vi "Graph_Settings.vi"() -> ()   [LabVIEW 2018]
uses:
  GraphSettings/GraphSettings_STM.ctl
  GraphSettings/GraphSettings_ITEM.ctl
  CTL/STM GRAPH.ctl
  CTL/Graph settings.ctl
  CTL/Line.ctl
  View.ctl
  <vilib>/Utility/miscctls.llb/LVComboBoxStrsAndValuesArrayTypeDef.ctl
  STM/Grafic/MOKO_Grafic_STM.ctl
  STM/Grafic/MOKO_Grafic_ITEM.ctl
panel:
  in  "Choice Line":string(combo) caption="Combo Box"
  in  "Color Box":u32(colorbox)
  in  "Delete":bool
  in  "Add Line":bool
  in  "Change Line":bool
  in  "Line":T1 {"Color" format="%x"}
  in  "Close":bool
  out "Flat UI Titlebar":bool
  in  "Settings":enum32{"Line", "Data"}(tab)
  in  "STM Graph":T3={"Graph settings"={"Axis X Min"=0.0, "Axis X Name"="", "Axis X Max"=0.0, "Axis Y Min"=0.0, " Axis Y Name"="", "Axis Y Max"=1.0, "Autoscale"=enum."Yes", "Choice Line"=1.0}, "Lines"=[], "Data"=""} {"Lines"."Color" format="%x"}
  out "Graph_Setting":refnum<queue>
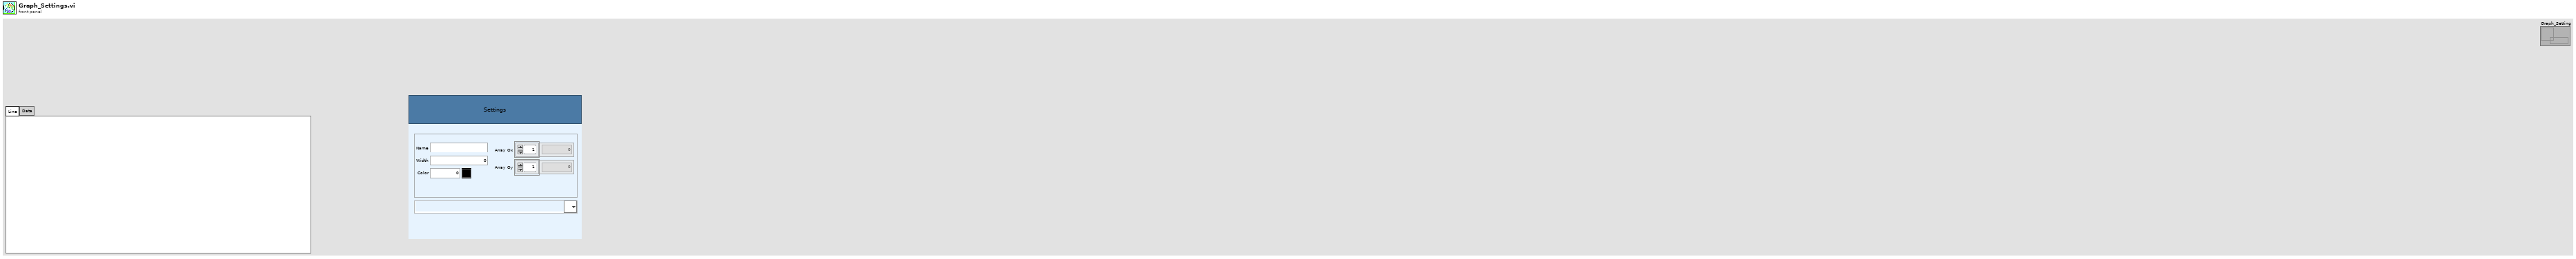
[diagram p1: front panel]
types:
  T1 = typedef "Line.ctl" = cluster{"Width":dbl, "Color":i64, "Array Oy":dbl[], "Array Ox":dbl[], "Name":string, "Plot Visible":T2}
  T2 = typedef "View.ctl" = bool
  T3 = typedef "STM GRAPH.ctl" = cluster{"Graph settings":T4, "Lines":T1[], "Data":string}
  T4 = typedef "Graph settings.ctl" = cluster{"Axis X Min":dbl, "Axis X Name":string, "Axis X Max":dbl, "Axis Y Min":dbl, " Axis Y Name":string, "Axis Y Max":dbl, "Autoscale":enum16{"Yes", "No", "Only Oy", "Only Ox"}, "Choice Line":dbl}
  T5 = typedef "GraphSettings_STM.ctl" = cluster{"main stm":T6, "STM Graph":T3}
  T6 = typedef "GraphSettings_ITEM.ctl" = enum16{"idle", "init", "close", "_____ GRAPH STATE_____ ", "Receive Data", "Send Data", "Change Line", "Delete Line", "Add Line", "Find Max", "Change Color", "Choice Line"}
  T7 = typedef "LVComboBoxStrsAndValuesArrayTypeDef.ctl" = cluster{"String":string, "Value":string}[]
  T8 = typedef "MOKO_Grafic_STM.ctl" = cluster{"main stm":T9, "STM Graph":T3}
  T9 = typedef "MOKO_Grafic_ITEM.ctl" = enum16{"idle", "init", "_____ GRAPH STATE_____ ", "Legend", "Write Graph", "Clear Graph", "close", "Screenshot", "Change Line", "Add Line", "Parse String In", "Add Data", "Change Data", "Graph Settings", "Get Graph Appearance", "Set Graph Appearance", "Delete Data", "Delete Line", "Choose ActPlot", "Set Line Settings", "Increment Smth", "ReWrite Graph", "Autoscale", "Set Autoscale", "Hide Line", "Get Hide Line", "Hide Data", "Show Line", "Get Show Line", "Show Data", "Choose Line", "Change Combo Box", "Send Data", "Receive Data", "Choice Line", "Change Lines", "_____ LED STATE_____ ", "Led Off"}
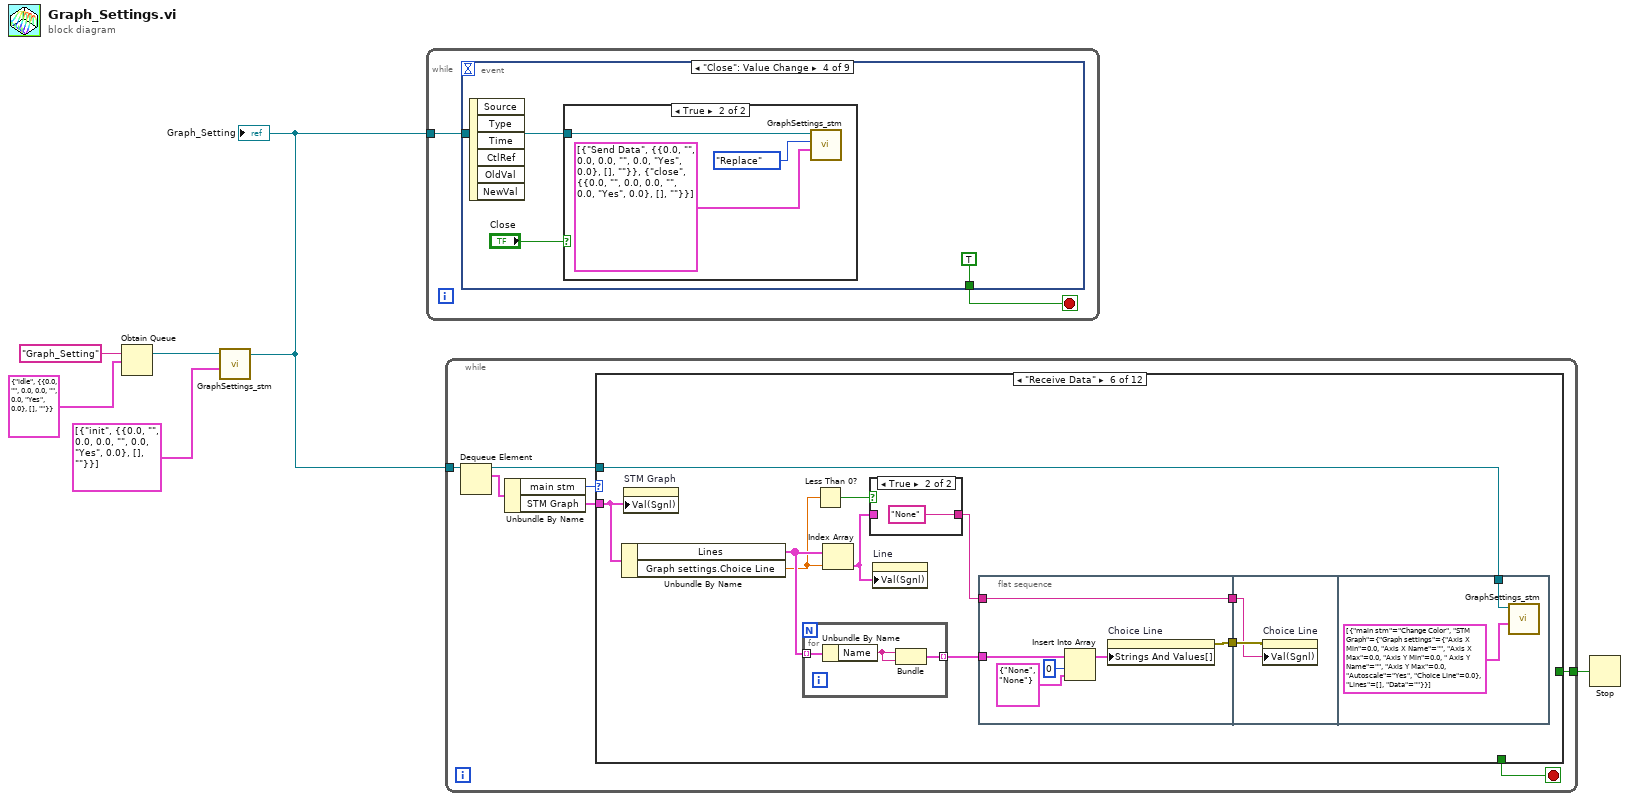
[diagram p0: block diagram]
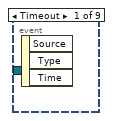
[diagram p2: hidden frame]
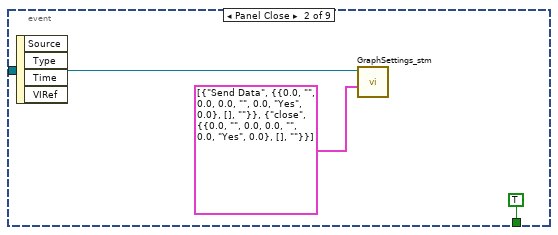
[diagram p3: hidden frame]
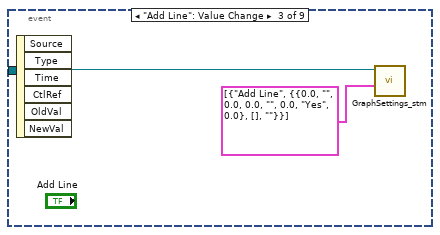
[diagram p4: hidden frame]
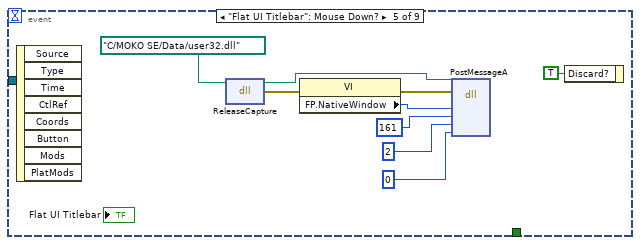
[diagram p6: hidden frame]
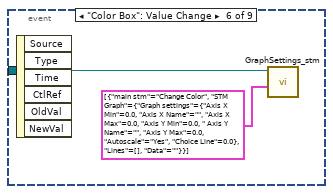
[diagram p7: hidden frame]
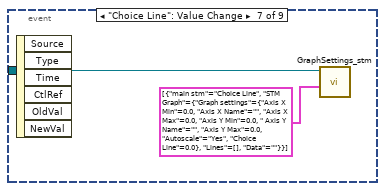
[diagram p8: hidden frame]
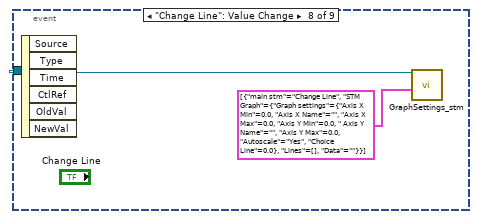
[diagram p9: hidden frame]
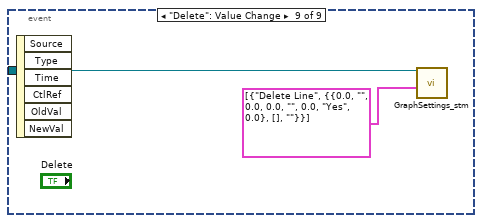
[diagram p10: hidden frame]
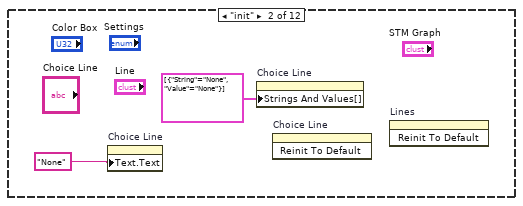
[diagram p16: hidden frame]
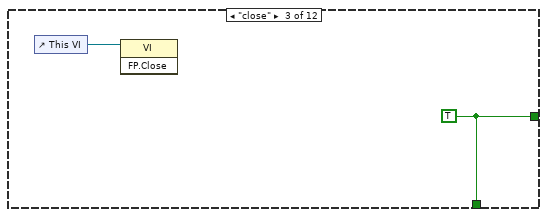
[diagram p17: hidden frame]
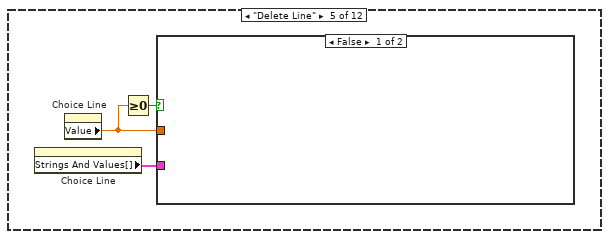
[diagram p19: hidden frame]
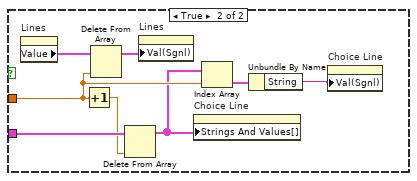
[diagram p20: hidden frame]
diagram:
  n1 = Obtain Queue(name (unnamed)="Graph_Setting", element data type=T5 {"main stm"=enum."idle", "STM Graph"={"Graph settings"={"Axis X Min"=0.0, "Axis X Name"="", "Axis X Max"=0.0, "Axis Y Min"=0.0, " Axis Y Name"="", "Axis Y Max"=0.0, "Autoscale"=enum."Yes", "Choice Line"=0.0}, "Lines"=[], "Data"=""}} ("MOKO_SE_STM")) -> (queue out=w5:refnum<queue>)  [unwired: 3 in, 2 out]
  n2 = call "GraphSettings_stm.vi"("StateMachineSteps"=T5[] [{"main stm"=enum."init", "STM Graph"={"Graph settings"={"Axis X Min"=0.0, "Axis X Name"="", "Axis X Max"=0.0, "Axis Y Min"=0.0, " Axis Y Name"="", "Axis Y Max"=0.0, "Autoscale"=enum."Yes", "Choice Line"=0.0}, "Lines"=[], "Data"=""}}], "queue in"=w5) -> ("queue out"=w3:refnum<queue>)  [unwired: 8 in, 1 out]
  "Graph_Setting" <- w3
  n3 = while {
    tunnel: w3 -> [w8]
    stop <- w7 stop-if-true
    n4 = event shown="[3] \"Close\": Value Change" {
      selector: _ -> [_ _ _ _ _ _ _ _ _]
      dyn-events: _ -> [_ _ _ _ _ _ _ _ _]
      timeout: _ -> [_ _ _ _ _ _ _ _ _]
      tunnel: w8 -> [_ w10 w12 w16 _ w29 w31 w33 w35]
      tunnel: [_ TRUE _ TRUE _ _ _ _ _] -> w7
      event Timeout {
        n5 = event-data() -> ()  [unwired: 1 in, 3 out]
      }
      event Panel Close {
        n6 = event-data() -> ()  [unwired: 1 in, 4 out]
        n7 = call "GraphSettings_stm.vi"("StateMachineSteps"=T5[] [{"main stm"=enum."Send Data", "STM Graph"={"Graph settings"={"Axis X Min"=0.0, "Axis X Name"="", "Axis X Max"=0.0, "Axis Y Min"=0.0, " Axis Y Name"="", "Axis Y Max"=0.0, "Autoscale"=enum."Yes", "Choice Line"=0.0}, "Lines"=[], "Data"=""}}, {"main stm"=enum."close", "STM Graph"={"Graph settings"={"Axis X Min"=0.0, "Axis X Name"="", "Axis X Max"=0.0, "Axis Y Min"=0.0, " Axis Y Name"="", "Axis Y Max"=0.0, "Autoscale"=enum."Yes", "Choice Line"=0.0}, "Lines"=[], "Data"=""}}], "queue in"=w10) -> ()  [unwired: 8 in, 2 out]
      }
      event "Add Line": Value Change {
        n8 = event-data() -> ()  [unwired: 1 in, 6 out]
        n9 = call "GraphSettings_stm.vi"("StateMachineSteps"=T5[] [{"main stm"=enum."Add Line", "STM Graph"={"Graph settings"={"Axis X Min"=0.0, "Axis X Name"="", "Axis X Max"=0.0, "Axis Y Min"=0.0, " Axis Y Name"="", "Axis Y Max"=0.0, "Autoscale"=enum."Yes", "Choice Line"=0.0}, "Lines"=[], "Data"=""}}], "queue in"=w12) -> ()  [unwired: 8 in, 2 out]
      }
      event "Close": Value Change {
        n10 = event-data() -> ()  [unwired: 1 in, 6 out]
        n11 = case shown="True" "Close" {
          tunnel: w16 -> [_ w19]
          frame False {
          }
          frame True {
            n12 = call "GraphSettings_stm.vi"("StateMachineSteps"=T5[] [{"main stm"=enum."Send Data", "STM Graph"={"Graph settings"={"Axis X Min"=0.0, "Axis X Name"="", "Axis X Max"=0.0, "Axis Y Min"=0.0, " Axis Y Name"="", "Axis Y Max"=0.0, "Autoscale"=enum."Yes", "Choice Line"=0.0}, "Lines"=[], "Data"=""}}, {"main stm"=enum."close", "STM Graph"={"Graph settings"={"Axis X Min"=0.0, "Axis X Name"="", "Axis X Max"=0.0, "Axis Y Min"=0.0, " Axis Y Name"="", "Axis Y Max"=0.0, "Autoscale"=enum."Yes", "Choice Line"=0.0}, "Lines"=[], "Data"=""}}], "FNs"=enum16{"Back", "Front", "Replace"}."Replace", "queue in"=w19) -> ()  [unwired: 7 in, 2 out]
          }
        }
      }
      event "Flat UI Titlebar": Mouse Down? {
        n13 = event-data() -> ()  [unwired: 1 in, 8 out]
        n14 = dll-call lib="C:/Windows/SysWOW64/user32.dll" fn="ReleaseCapture"(path in=path "C:/MOKO SE/Data/user32.dll") -> (path out=w20:path, error out=w27:errorcluster)  [unwired: 3 in]
        n15 = property class="VI"(error in=w27) -> (error out=w26:errorcluster, "FP.NativeWindow"=w25:u64)  [unwired: 1 in, 1 out]
        n16 = dll-call lib="C:/Windows/SysWOW64/user32.dll" fn="PostMessageA"(path in=w20, error in=w26, "hWnd"=w25, "Msg"=161, "wParam"=2, "lParam"=0) -> ()  [unwired: 6 in, 2 out]
        n17 = event-data("Discard?"=TRUE) -> ()  [unwired: 1 in, 1 out]
      }
      event "Color Box": Value Change {
        n18 = event-data() -> ()  [unwired: 1 in, 6 out]
        n19 = call "GraphSettings_stm.vi"("StateMachineSteps"=T5[] [{"main stm"=enum."Change Color", "STM Graph"={"Graph settings"={"Axis X Min"=0.0, "Axis X Name"="", "Axis X Max"=0.0, "Axis Y Min"=0.0, " Axis Y Name"="", "Axis Y Max"=0.0, "Autoscale"=enum."Yes", "Choice Line"=0.0}, "Lines"=[], "Data"=""}}], "queue in"=w29) -> ()  [unwired: 8 in, 2 out]
      }
      event "Choice Line": Value Change {
        n20 = event-data() -> ()  [unwired: 1 in, 6 out]
        n21 = call "GraphSettings_stm.vi"("StateMachineSteps"=T5[] [{"main stm"=enum."Choice Line", "STM Graph"={"Graph settings"={"Axis X Min"=0.0, "Axis X Name"="", "Axis X Max"=0.0, "Axis Y Min"=0.0, " Axis Y Name"="", "Axis Y Max"=0.0, "Autoscale"=enum."Yes", "Choice Line"=0.0}, "Lines"=[], "Data"=""}}], "queue in"=w31) -> ()  [unwired: 8 in, 2 out]
      }
      event "Change Line": Value Change {
        n22 = event-data() -> ()  [unwired: 1 in, 6 out]
        n23 = call "GraphSettings_stm.vi"("StateMachineSteps"=T5[] [{"main stm"=enum."Change Line", "STM Graph"={"Graph settings"={"Axis X Min"=0.0, "Axis X Name"="", "Axis X Max"=0.0, "Axis Y Min"=0.0, " Axis Y Name"="", "Axis Y Max"=0.0, "Autoscale"=enum."Yes", "Choice Line"=0.0}, "Lines"=[], "Data"=""}}], "queue in"=w33) -> ()  [unwired: 8 in, 2 out]
      }
      event "Delete": Value Change {
        n24 = event-data() -> ()  [unwired: 1 in, 6 out]
        n25 = call "GraphSettings_stm.vi"("StateMachineSteps"=T5[] [{"main stm"=enum."Delete Line", "STM Graph"={"Graph settings"={"Axis X Min"=0.0, "Axis X Name"="", "Axis X Max"=0.0, "Axis Y Min"=0.0, " Axis Y Name"="", "Axis Y Max"=0.0, "Autoscale"=enum."Yes", "Choice Line"=0.0}, "Lines"=[], "Data"=""}}], "queue in"=w35) -> ()  [unwired: 8 in, 2 out]
      }
    }
  }
  n26 = while {
    tunnel: w3 -> [w43]
    tunnel: [w37] -> w1
    stop <- w39 stop-if-true
    n27 = Dequeue Element(queue=w43) -> (queue out=w42:refnum<queue>, element=w40:T5)  [unwired: 2 in, 2 out]
    n28 = Unbundle By Name(w40) -> ("main stm"=w41:T6, "STM Graph"=w38:T3)
    n29 = case shown="\"Receive Data\"" w41 {
      tunnel: w42 -> [_ _ _ _ _ w60 _ _ _ _ _ _]
      tunnel: w38 -> [_ _ _ _ _ w59 _ _ _ _ _ _]
      tunnel: [_ _ w47 _ _ _ _ _ _ _ _ _] -> w39
      tunnel: [_ _ w47 _ _ _ _ _ _ _ _ _] -> w37
      frame "idle", Default {
        n30 = stacked-sequence {
          frame #0 {
            # "Удаление графика:\nВ скрипте:\n    1. Выбрать имя плагина\n    2. Выбрать set\n    3. Выбрать команду\n    4. Передать номер графика\nПример команды в скрипте:\nnumLine = 3\nMOKO.Plugin(\"MOKO Graph\", 'set', 'Delete Line', numLine)\n\nВ LabView:\n1. Принять данные\n2. Удалить в кластере\n3. Удалить в Array Graphs\n4. Отобразить на графике"
          }
          frame #1 {
            # "Изменение графика:\nВ скрипте:\n    1. Выбрать имя плагина\n    2. Выбрать set\n    3. Выбрать команду\n    4. Передать все параметры графика\nВозможно, между данными нужно ставить \";\", чтобы потом их разделить в LabView\nПример команды в скрипте:\nnumLine = 1\nLineWidth = 1\nColor = 'Blue'\nArrOx = {1,2,3,4}\nArrOy = {1,2,35,6}\nMOKO.Plugin(\"MOKO Graph\", 'set', 'Change Line', numLine + ArrOx + ArrOy + LineWidth+Color)\n\nВ LabView:\n1. Принять и разделить данные\n2. Заменить в кластере старые значения на новые\n2. Найти старый массив в Array Graphs и заменить на новый"
          }
          frame #2 {
            # "Изменение подписей, и min, и max для осей:\nВ скрипте:\n    1. Выбрать имя плагина\n    2. Выбрать set\n    3. Выбрать команду\n    4. Передать параметры\nВозможно, между данными нужно ставить \";\", чтобы потом их разделить в LabView\nПример команды в скрипте:\nYmax = 5; Ymin = 0\nXmax = 5; Xmin = 0\nName Oy = \"Amplitude\"\nName Ox = \"Frequency\"\nMOKO.Plugin(\"MOKO Graph\", 'set', 'Change Придумать команду', Ymax+Ymin+Xmax+Xmin+NameOy+NameOx)\n\nВ LabView:\n1. Принять и разделить данные\n2. Изменить в кластере\n3. Отобразить на графике"
          }
          frame #3 {
            # "Добавление графика:\nВ скрипте:\n    1. Выбрать имя плагина\n    2. Выбрать set\n    3. Выбрать команду\n    4. Передать параметры графика\nВозможно, между данными нужно ставить \";\", чтобы потом их разделить в LabView\nПример команды в скрипте:\nnumLine = 1\nColor = 'Red'\nLineWidth = 1\nArrOx = {1,2,3,4}\nArrOy = {1,2,35,6}\nMOKO.Plugin(\"MOKO Graph\", 'set', 'Add Line', ArrOx + ArrOy + LineWidth + Color)\nНомер графика передавать не нужно, потому что LabView будет вести индексацию\n\nВ LabView:\n1. Принять и разделить данные\n2. Записать в кластер\n3. Добавить в Array Graphs\n4. Отобразить на графике"
          }
          frame #4 {
            # "Добавление подписей, и min, и max для осей:\nВ скрипте:\n    1. Выбрать имя плагина\n    2. Выбрать set\n    3. Выбрать команду\n    4. Передать параметры\nВозможно, между данными нужно ставить \";\", чтобы потом их разделить в LabView\nПример команды в скрипте:\nValue_OyOx = {0,5,0,4}\nName_OyOx = {\"Ampl\", \"Freq\"}\nMOKO.Plugin(\"MOKO Graph\", 'set', 'Add Придумать команду', f\"{Value_OyOx};{Name_OyOx})\n\nВ LabView:\n1. Принять и разделить данные\n2. Записать в кластер\n3. Отобразить на графике"
          }
        }
      }
      frame "init" {
        n31 = property on="Choice Line" class="CmbBox"("Text.Text"="None") -> ()  [unwired: 2 in, 2 out]
        n32 = property on="Choice Line" class="CmbBox"("Strings And Values[]"=T7 [{"String"="None", "Value"="None"}] ("Strings And Values []")) -> ()  [unwired: 2 in, 2 out]
        n33 = invoke on="Choice Line" class="DigNum (strict)" method="Reinit To Default"() -> ()  [unwired: 3 in, 3 out]
        n34 = invoke on="Lines" class="Arr (strict)" method="Reinit To Default"() -> ()  [unwired: 3 in, 3 out]
      }
      frame "close" {
        w47 = TRUE
        n35 = control-ref of="This VI"() -> (w46:refnum<vi>)
        n36 = invoke class="VI" method="FP.Close"(reference=w46) -> ()  [unwired: 2 in, 3 out]
      }
      frame "_____ GRAPH STATE_____ " {
      }
      frame "Delete Line" {
        n37 = property on="Choice Line" class="CmbBox"() -> ("Strings And Values[]"=w48:T7)  [unwired: 2 in, 2 out]
        n38 = property on="Choice Line" class="DigNum (strict)"() -> ("Value"=w49:dbl)  [unwired: 2 in, 2 out]
        n39 = Greater Or Equal To 0?(x=w49) -> (x >= 0?=w50:bool)
        n40 = case shown="False" w50 {
          tunnel: w48 -> [_ w56]
          tunnel: w49 -> [_ w53]
          frame False {
          }
          frame True {
            n41 = property on="Lines" class="Arr (strict)"() -> ("Value"=w58:T1[])  [unwired: 2 in, 2 out]
            n42 = Increment(x=w53) -> (x+1=w55:dbl)
            n43 = Delete From Array(array=w58, index=w53) -> (array with subset deleted=w57:T1[])  [unwired: 1 in, 1 out]
            n44 = Delete From Array(array=w56, index=w55) -> (array with subset deleted=w52:T7)  [unwired: 1 in, 1 out]
            n45 = property on="Lines" class="Arr (strict)"("Val(Sgnl)"=w57) -> ()  [unwired: 2 in, 2 out]
            n46 = property on="Choice Line" class="CmbBox"("Strings And Values[]"=w52) -> ()  [unwired: 2 in, 2 out]
            n47 = Index Array(array=w52, index=w53) -> (element=w54:cluster{"String":string, "Value":string})
            n48 = Unbundle By Name(w54) -> ("String"=w51:string)
            n49 = property on="Choice Line" class="CmbBox"("Val(Sgnl)"=w51) -> ()  [unwired: 2 in, 2 out]
          }
        }
      }
      frame "Receive Data" {
        n50 = Unbundle By Name(w59) -> ("Lines"=w68:T1[], "Graph settings.Choice Line"=w63:dbl)
        n51 = property on="STM Graph" class="Clust (strict)"("Val(Sgnl)"=w59) -> ()  [unwired: 2 in, 2 out]
        n52 = for {
          tunnel: w68 -> [w84] mode=indexing
          tunnel: [w82] -> w67 mode=indexing
          n53 = Unbundle By Name(w84) -> ("Name"=w83:string)
          n54 = Bundle("Name"=w83, "Name"=w83) -> (w82:cluster{"Name":string, "Name":string})  [unwired: 1 in]
        }
        n55 = Less Than 0?(x=w63) -> (x < 0?=w64:bool)
        n56 = Index Array(array=w68, index=w63) -> (element=w62:T1)
        n57 = case shown="True" w64 {
          tunnel: w62 -> [w70 _]
          tunnel: [w69 "None" ("Name")] -> w61
          frame False {
            n58 = Unbundle By Name(w70) -> ("Name"=w69:string)
          }
          frame True {
          }
        }
        n59 = property on="Line" class="Clust (strict)"("Val(Sgnl)"=w62) -> ()  [unwired: 2 in, 2 out]
        n60 = flat-sequence {
          tunnel: w67 -> [w76]
          tunnel: [w72] -> w66
          tunnel: w61 -> [w74]
          tunnel: [w74] -> w65
          tunnel: w66 -> [w79]
          tunnel: w65 -> [w78]
          tunnel: w60 -> [w80]
          frame #0 {
            n61 = Insert Into Array(array=w76, index=0, new element=cluster{"Name":string, "Name":string} {"Name"="None", "Name"="None"} ("new element/subarray")) -> (w73:cluster{"Name":string, "Name":string}[])
            n62 = property on="Choice Line" class="CmbBox"("Strings And Values[]"=w73) -> (error out=w72:errorcluster)  [unwired: 2 in, 1 out]
          }
          frame #1 {
            n63 = property on="Choice Line" class="CmbBox"(error in=w79, "Val(Sgnl)"=w78) -> ()  [unwired: 1 in, 2 out]
          }
          frame #2 {
            n64 = call "GraphSettings_stm.vi"("StateMachineSteps"=T5[] [{"main stm"=enum."Change Color", "STM Graph"={"Graph settings"={"Axis X Min"=0.0, "Axis X Name"="", "Axis X Max"=0.0, "Axis Y Min"=0.0, " Axis Y Name"="", "Axis Y Max"=0.0, "Autoscale"=enum."Yes", "Choice Line"=0.0}, "Lines"=[], "Data"=""}}], "queue in"=w80) -> ()  [unwired: 8 in, 2 out]
          }
        }
      }
      frame "Send Data" {
        n65 = property on="STM Graph" class="Clust (strict)"() -> ("Value"=w88:T3)  [unwired: 2 in, 2 out]
        n66 = Bundle By Name(cluster=T8 {"main stm"=enum."Receive Data", "STM Graph"={"Graph settings"={"Axis X Min"=0.0, "Axis X Name"="", "Axis X Max"=0.0, "Axis Y Min"=0.0, " Axis Y Name"="", "Axis Y Max"=0.0, "Autoscale"=enum."Yes", "Choice Line"=0.0}, "Lines"=[], "Data"=""}} ("MOKO_SE_STM"), "STM Graph"=w88) -> (w89:T8)
        n67 = vi-ref "MOKO Graph.vi"() -> (w85:refnum<vi>)
        n68 = call "OpenAndSendDataToMainVi(SubVI).vi"("reference"=w85, "Control Name"="MOKO_GRAPH_STM", "element"=w89) -> ()  [unwired: 8 in]
      }
      frame "Change Line" {
        n69 = property on="Choice Line" class="DigNum (strict)"() -> ("Value"=w90:dbl)  [unwired: 2 in, 2 out]
        n70 = Greater Or Equal To 0?(x=w90) -> (x >= 0?=w91:bool)
        n71 = case shown="True" w91 {
          tunnel: w90 -> [_ w107]
          frame False {
          }
          frame True {
            w99 = 5.0 ("y")
            n72 = property on="Line" class="Clust (strict)"() -> ("Value"=w117:T1)  [unwired: 2 in, 2 out]
            n73 = property on="Lines" class="Arr (strict)"() -> ("Value"=w108:T1[])  [unwired: 2 in, 2 out]
            n74 = Unbundle By Name(w117) -> ("Name"=w103:string, "Array Oy"=w115:dbl[], "Array Ox"=w114:dbl[], "Width"=w98:dbl, "Color"=w112:i64, "Plot Visible"=w113:T2)
            n75 = Index Array(array=w108, index=w107) -> (element=w106:T1)
            n76 = property on="Choice Line" class="CmbBox"() -> ("Strings And Values[]"=w95:T7)  [unwired: 2 in, 2 out]
            n77 = Unbundle By Name(w106) -> ("Name"=w104:string)
            n78 = Greater?(x=w98, y=w99) -> (0:w100:bool)
            n79 = Equal?(x=w104, y=w103) -> (x = y?=w105:bool)
            n80 = case shown="True" w100 {
              tunnel: w99 -> [_ w119]
              tunnel: w98 -> [w118 _]
              tunnel: [w118 w119] -> w97
              frame False {
              }
              frame True {
              }
            }
            n81 = case shown="False" w105 {
              tunnel: w103 -> [w122 w123]
              tunnel: w95 -> [w121 _]
              tunnel: [w120 w123] -> w94
              frame False {
                n82 = call "CheckName(SubVI).vi"("Name In"=w122, "Strings And Values[]"=w121) -> ("Name Out"=w120:string)  [unwired: 8 in, 1 out]
              }
              frame True {
              }
            }
            n83 = property on="Line" class="Clust (strict)"() -> ("Value"=w116:T1)  [unwired: 2 in, 2 out]
            n84 = Bundle By Name(cluster=w116, "Name"=w94, "Array Oy"=w115, "Array Ox"=w114, "Width"=w97, "Color"=w112, "Plot Visible"=w113) -> (w96:T1)
            n85 = property on="Choice Line" class="CmbBox"() -> ("Strings And Values[]"=w93:T7)  [unwired: 2 in, 2 out]
            n86 = property on="Choice Line" class="CmbBox"("Text.Text"=w94) -> ()  [unwired: 2 in, 2 out]
            n87 = property on="Lines" class="Arr (strict)"() -> ("Value"=w111:T1[])  [unwired: 2 in, 2 out]
            n88 = property on="Choice Line" class="DigNum (strict)"() -> ("Value"=w102:dbl)  [unwired: 2 in, 2 out]
            n89 = Bundle("Name"=w94, "Name"=w94) -> (w109:cluster{"Name":string, "Name":string})  [unwired: 1 in]
            n90 = Increment(x=w102) -> (x+1=w101:dbl)
            n91 = Replace Array Subset(array=w111, new element=w96, index=w102) -> (w110:T1[])
            n92 = property on="Line" class="Clust (strict)"("Val(Sgnl)"=w96) -> ()  [unwired: 2 in, 2 out]
            n93 = Replace Array Subset(array=w93, new element=w109, index=w101) -> (w92:T7)
            n94 = property on="Lines" class="Arr (strict)"("Val(Sgnl)"=w110) -> ()  [unwired: 2 in, 2 out]
            n95 = property on="Choice Line" class="CmbBox"("Strings And Values[]"=w92) -> ()  [unwired: 2 in, 2 out]
          }
        }
      }
      frame "Change Color" {
        n96 = property on="Line" class="Clust (strict)"() -> ("Value"=w131:T1)  [unwired: 2 in, 2 out]
        n97 = Unbundle By Name(w131) -> ("Name"=w130:string, "Array Oy"=w129:dbl[], "Array Ox"=w128:dbl[], "Width"=w127:dbl, "Plot Visible"=w125:T2)
        n98 = property on="Color Box" class="ColBox"() -> ("Value"=w124:u32)  [unwired: 2 in, 2 out]
        n99 = Bundle By Name(cluster=w131, "Name"=w130, "Array Oy"=w129, "Array Ox"=w128, "Width"=w127, "Plot Visible"=w125, "Color"=w124) -> (w126:T1)
        n100 = property on="Line" class="Clust (strict)"("Val(Sgnl)"=w126) -> ()  [unwired: 2 in, 2 out]
      }
      frame "Add Line" {
        w137 = 5.0 ("y")
        n101 = property on="Choice Line" class="CmbBox"() -> ("Strings And Values[]"=w134:T7)  [unwired: 2 in, 2 out]
        n102 = property on="Line" class="Clust (strict)"() -> ("Value"=w146:T1)  [unwired: 2 in, 2 out]
        n103 = Unbundle By Name(w146) -> ("Name"=w152:string, "Array Oy"=w151:dbl[], "Array Ox"=w150:dbl[], "Width"=w135:dbl, "Color"=w148:i64, "Plot Visible"=w149:T2)
        n104 = Greater?(x=w135, y=w137) -> (0:w138:bool)
        n105 = case shown="False" w138 {
          tunnel: w137 -> [_ w154]
          tunnel: [w153 w154] -> w136
          tunnel: w135 -> [w153 _]
          frame False {
          }
          frame True {
          }
        }
        n106 = call "CheckName(SubVI).vi"("Name In"=w152, "Strings And Values[]"=w134) -> ("Name Out"=w142:string)  [unwired: 8 in, 1 out]
        n107 = property on="Line" class="Clust (strict)"() -> ("Value"=w145:T1)  [unwired: 2 in, 2 out]
        n108 = Bundle By Name(cluster=w145, "Name"=w142, "Array Oy"=w151, "Array Ox"=w150, "Width"=w136, "Color"=w148, "Plot Visible"=w149) -> (w147:T1)
        n109 = property on="Lines" class="Arr (strict)"() -> ("Value"=w143:T1[])  [unwired: 2 in, 2 out]
        n110 = property on="Choice Line" class="CmbBox"() -> ("Strings And Values[]"=w133:T7)  [unwired: 2 in, 2 out]
        n111 = Bundle("Name Out"=w142, "Name Out"=w142) -> (w141:cluster{"Name Out":string, "Name Out":string})  [unwired: 1 in]
        n112 = Array Size(array=w143) -> (size(s)=w140:i32)
        n113 = Increment(x=w140) -> (x+1=w139:i32)
        n114 = Insert Into Array(array=w143, index=w140, new element=w147) -> (w144:T1[])
        n115 = Insert Into Array(array=w133, index=w139, new element=w141) -> (w132:T7)
        n116 = property on="Lines" class="Arr (strict)"("Val(Sgnl)"=w144) -> ()  [unwired: 2 in, 2 out]
        n117 = property on="Choice Line" class="CmbBox"("Strings And Values[]"=w132) -> ()  [unwired: 2 in, 2 out]
      }
      frame "Choice Line" {
        n118 = property on="Choice Line" class="CmbBox"() -> ("Strings And Values[]"=w156:T7)  [unwired: 2 in, 2 out]
        n119 = property on="Choice Line" class="CmbBox"() -> ("Text.Text"=w155:string)  [unwired: 2 in, 2 out]
        n120 = Index Array(array=w156, index=0) -> (element=w159:cluster{"String":string, "Value":string})
        n121 = Unbundle By Name(w159) -> ("String"=w158:string)
        n122 = Not Equal?(x=w158, y=w155) -> (x != y?=w157:bool)
        n123 = case shown="False" w157 {
          tunnel: w156 -> [_ w168]
          tunnel: w155 -> [_ w167]
          frame False {
            n124 = property on="Choice Line" class="DigNum (strict)"("Val(Sgnl)"=-1.0 ("Value (Signaling)")) -> ()  [unwired: 2 in, 2 out]
          }
          frame True {
            n125 = while {
              tunnel: w168 -> [w174]
              tunnel: w167 -> [w172]
              tunnel: [w169] -> w164
              i -> [w169]
              stop <- w173 stop-if-true
              n126 = Index Array(array=w174, index=w169) -> (element=w171:cluster{"String":string, "Value":string})
              n127 = Unbundle By Name(w171) -> ("String"=w170:string)
              n128 = Equal?(x=w170, y=w172) -> (x = y?=w173:bool)
            }
            n129 = property on="Lines" class="Arr (strict)"() -> ("Value"=w166:T1[])  [unwired: 2 in, 2 out]
            n130 = Decrement(x=w164) -> (x-1=w163:i32)
            n131 = Index Array(array=w166, index=w163) -> (element=w165:T1)
            n132 = property on="Choice Line" class="DigNum (strict)"("Val(Sgnl)"=w163) -> ()  [unwired: 2 in, 2 out]
            n133 = property on="Line" class="Clust (strict)"("Val(Sgnl)"=w165) -> ()  [unwired: 2 in, 2 out]
            n134 = Unbundle By Name(w165) -> ("Color"=w162:i64)
            n135 = property on="Color Box" class="ColBox"("Value"=w162) -> ()  [unwired: 2 in, 2 out]
          }
        }
      }
      frame "Find Max" {
        n136 = disable-structure shown="Disabled" {
          frame Disabled {
            n137 = flat-sequence {
              tunnel: [w180] -> w176
              tunnel: [w179] -> w175
              tunnel: w176 -> [w184]
              tunnel: w175 -> [w183]
              frame #0 {
                (unwired) TRUE ("Value (Signaling)")
                # "Индикатор"
              }
              frame #1 {
                # "Позиция курсора по Ох"
                # "Позиция курсора по Оу"
                n138 = Array Max & Min(array=dbl[] []) -> (max value=w180:dbl, max index (indices)=w181:i32)  [unwired: 2 out]
                n139 = Index Array(array=dbl[] [], index=w181) -> (element=w179:dbl)
                n140 = Build Array(w180, w179) -> (w182:dbl[])
                n141 = call "ArrayIntoString(SubVI).vi"("Array"=w182) -> ()  [unwired: 1 out]
              }
              frame #2 {
                (unwired) FALSE ("Value (Signaling)")
                # "Индикатор"
                n142 = call "ChangeDoubleValue(SubVI).vi"("numbers after decimal point"=2.0, "NumIn"=w184) -> ()  [unwired: 1 out]
                n143 = call "ChangeDoubleValue(SubVI).vi"("numbers after decimal point"=2.0, "NumIn"=w183) -> ()  [unwired: 1 out]
              }
            }
          }
          frame Enabled {
          }
        }
      }
    }
  }
  n144 = Stop(stop? (T)=w1) -> ()
